vi "Get Dependency State Events.vi"(8 "error in (no error)":errorcluster, 11 "SMO in":refnum<class "SMO.lvclass">) -> (0 "error out":errorcluster, 1 "Error [Dependencies]":refnum<user-event>[](array[refnum]), 2 "State [Dependencies]":refnum<user-event>[](array[refnum]), 3 "SMO out":refnum<class "SMO.lvclass">, 4 "Message [Dependencies]":refnum<user-event>[](array[refnum]), 5 "[Dependencies]":refnum<class "SMO.lvclass">[](array[class]))   [LabVIEW 2013, in "SMO.lvclass"]
uses:
  SMO.lvclass
  Typedefs/SMOState --Enum.ctl
  Support/Attribute.Owner/Packet -- Cluster.ctl
  SMO.lvclass/SMO.ctl
  Support/Attribute.Owner/Attribute.Owner.lvclass/Attribute.Owner.ctl
  Private/GetDependencies.vi
  Support/Attribute.Dependencies/List Dependencies.vi
  Private/GetVariant(Attr).vi
  Private/ReftoDVR--SMO.vi
  Support/Attribute.Dependencies/Get GUIDs.vi
  isStateMachineObject.vi
  Support/Attribute.Dependencies/Attribute.Dependencies.lvclass
  Support/Attribute.Owner/Attribute.Owner.lvclass
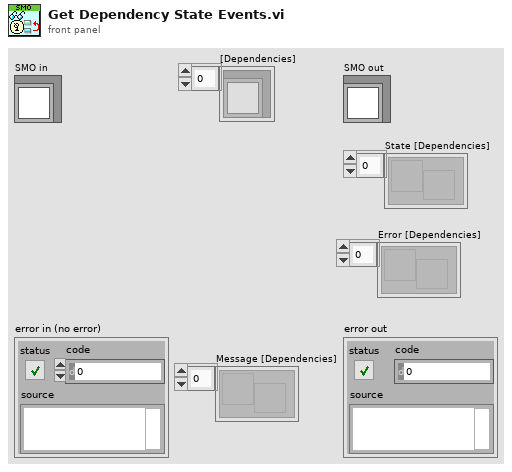
[diagram p1: front panel]
types:
  T1 = typedef "SMO.lvclass/Public Events.ctl" = cluster{"Error":refnum<user-event>, "State":refnum<user-event>, "Reserve State":refnum<user-event>}
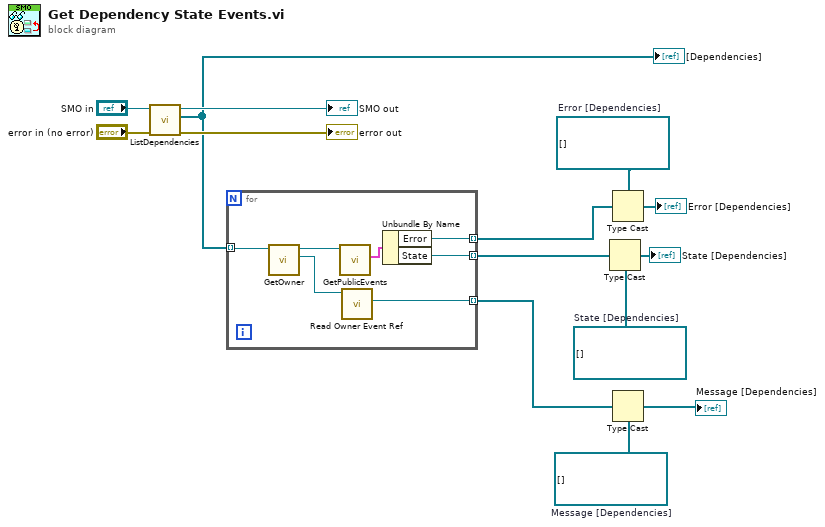
[diagram p0: block diagram]
diagram:
  w3 = refnum<user-event>[] []  # Message [Dependencies]
  w4 = refnum<user-event>[] []  # Error [Dependencies]
  w12 = refnum<user-event>[] [] items=["unknown", "Created", "Started", "Stopped"]  # State [Dependencies]
  n1 = call "ListDependencies.vi"("error in (no error)"="error in (no error)", "SMO in"="SMO in") -> ("error out"=→"error out":errorcluster, "[Dependencies]"=w7:refnum<class "SMO.lvclass">[], "SMO out"=→"SMO out":refnum<class "SMO.lvclass">)  [unwired: 6 in, 1 out]
  "[Dependencies]" <- w7
  n2 = for {
    tunnel: w7 -> [w17] mode=indexing
    tunnel: [w20] -> w13 mode=indexing
    tunnel: [w19] -> w6 mode=indexing
    tunnel: [w18] -> w1 mode=indexing
    n3 = call "GetOwner.vi"("SMO in"=w17) -> ("Owner"=w15:refnum<class "Attribute.Owner.lvclass">, "SMO out"=w16:refnum<class "SMO.lvclass">)  [unwired: 7 in, 2 out]
    n4 = call "GetPublicEvents.vi"("SMO"=w16) -> ("Public Events"=w21:T1)  [unwired: 8 in, 2 out]
    n5 = call "Read Owner Event Ref.vi"("Attribute.Owner in"=w15) -> ("Upstream Ref"=w18:refnum<user-event>)  [unwired: 8 in, 2 out]
    n6 = Unbundle By Name(w21) -> ("Error"=w19:refnum<user-event>, "State"=w20:refnum<user-event>)
  }
  n7 = Type Cast(type=w12, x=w13) -> (*(type *) &x=→"State [Dependencies]":refnum<user-event>[])
  n8 = Type Cast(type=w4, x=w6) -> (*(type *) &x=→"Error [Dependencies]":refnum<user-event>[])
  n9 = Type Cast(type=w3, x=w1) -> (*(type *) &x=→"Message [Dependencies]":refnum<user-event>[])
